vi "HMI_quadrant.vi"() -> ()   [LabVIEW 2019]
panel:
  out "output variable":i16
  in  "y":dbl
  in  "x":dbl
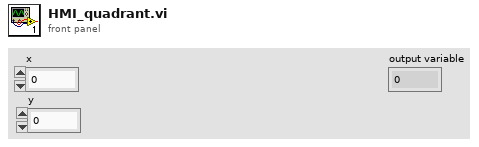
[diagram p1: front panel]
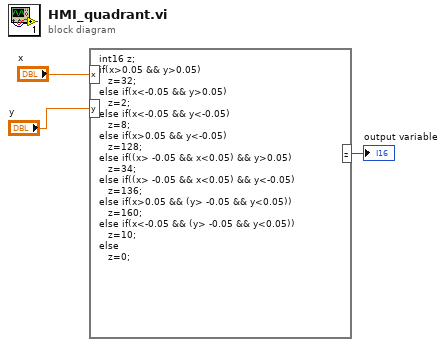
[diagram p0: block diagram]
diagram:
  n1 = formula code="int16 z;\nif(x>0.05 && y>0.05)\n   z=32;\nelse if(x<-0.05 && y>0.05)\n   z=2;\nelse if(x<-0.05 && y<-0.05)\n   z=8;\nelse if(x>0.05 && y<-0.05)\n   z=128;\nelse if((x> -0.05 && x<0.05) && y>0.05)\n   z=34;\nelse if((x> -0.05 && x<0.05) && y<-0.05)\n   z=136;\nelse if(x>0.05 && (y> -0.05 && y<0.05))\n   z=160;\nelse if(x<-0.05 && (y> -0.05 && y<0.05))\n   z=10;\nelse\n   z=0;"("x"="x", "y"="y") -> ("z"=→"output variable":i16)
